vi "PathPlanner_Trajectory_CalculateVelocity.vi"(9 "MaxAccel":dbl, 10 "PathPoints":T1[](array[typedef]) {"HolonomicRotation"."SIN" format="%13.4f"; "HolonomicRotation"."COS" format="%13.4f"; "HolonomicRotation"."VALUE" format="%13.4f"; "NextControl"."Y" format="%14.3f"; "NextControl"."X" format="%14.3f"; "PrevControl"."Y" format="%14.3f"; "PrevControl"."X" format="%14.3f"; "AnchorPoint"."Y" format="%14.3f"; "AnchorPoint"."X" format="%14.3f"}, 11 "PathPlannerStates":T4[](array[typedef]) {"HolonomicRotation"."SIN" format="%13.4f"; "HolonomicRotation"."COS" format="%13.4f"; "HolonomicRotation"."VALUE" format="%13.4f"; "AngularVelocity"."SIN" format="%13.4f"; "AngularVelocity"."COS" format="%13.4f"; "AngularVelocity"."VALUE" format="%13.4f"; "TrajectoryState"."POSE"."ROTATION"."SIN" format="%13.4f"; "TrajectoryState"."POSE"."ROTATION"."COS" format="%13.4f"; "TrajectoryState"."POSE"."ROTATION"."VALUE" format="%13.4f"; "TrajectoryState"."POSE"."TRANSLATION"."Y" format="%14.3f"; "TrajectoryState"."POSE"."TRANSLATION"."X" format="%14.3f"; "AngularAcceleration"."SIN" format="%13.4f"; "AngularAcceleration"."COS" format="%13.4f"; "AngularAcceleration"."VALUE" format="%13.4f"}) -> (3 "outPathPlannerStates":T4[](array[typedef]) {"HolonomicRotation"."SIN" format="%13.4f"; "HolonomicRotation"."COS" format="%13.4f"; "HolonomicRotation"."VALUE" format="%13.4f"; "AngularVelocity"."SIN" format="%13.4f"; "AngularVelocity"."COS" format="%13.4f"; "AngularVelocity"."VALUE" format="%13.4f"; "TrajectoryState"."POSE"."ROTATION"."SIN" format="%13.4f"; "TrajectoryState"."POSE"."ROTATION"."COS" format="%13.4f"; "TrajectoryState"."POSE"."ROTATION"."VALUE" format="%13.4f"; "TrajectoryState"."POSE"."TRANSLATION"."Y" format="%14.3f"; "TrajectoryState"."POSE"."TRANSLATION"."X" format="%14.3f"; "AngularAcceleration"."SIN" format="%13.4f"; "AngularAcceleration"."COS" format="%13.4f"; "AngularAcceleration"."VALUE" format="%13.4f"})   [LabVIEW 2019, in "PathPlanner.lvlib"]
uses:
  PathPlanner.lvlib
  PathPlannerState.ctl
  <vilib>/Rock Robotics/WPI/ThirdParty/JAS_Junk/TrajLib/ROTATION2D.ctl
  <vilib>/Rock Robotics/WPI/ThirdParty/JAS_Junk/TrajLib/TRAJ_STATE.ctl
  <vilib>/Rock Robotics/WPI/ThirdParty/JAS_Junk/TrajLib/POSE2D.ctl
  <vilib>/Rock Robotics/WPI/ThirdParty/JAS_Junk/TrajLib/TRANSLATION2D.ctl
  PathPlannerWaypoint.ctl
  <vilib>/Rock Robotics/WPI/ThirdParty/JAS_Junk/TrajLib/Trajectory_Library.lvlib
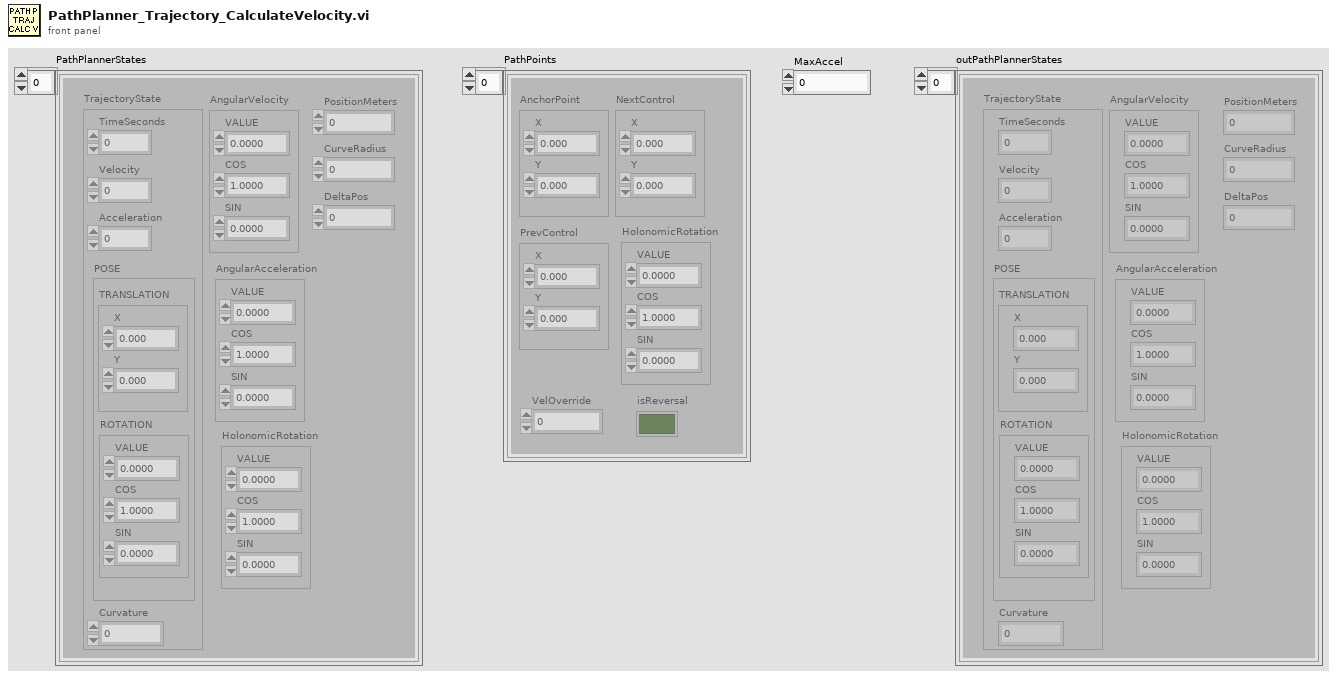
[diagram p1: front panel]
types:
  T1 = typedef "PathPlanner.lvlib/PathPlannerWaypoint.ctl" = cluster{"AnchorPoint":T2, "PrevControl":T2, "NextControl":T2, "HolonomicRotation":T3, "VelOverride":dbl, "isReversal":bool}
  T2 = typedef "Trajectory_Library.lvlib/TRANSLATION2D.ctl" = cluster{"X":dbl, "Y":dbl}
  T3 = typedef "Trajectory_Library.lvlib/ROTATION2D.ctl" = cluster{"VALUE":dbl, "COS":dbl, "SIN":dbl}
  T4 = typedef "PathPlanner.lvlib/PathPlannerState.ctl" = cluster{"AngularAcceleration":T3, "PositionMeters":dbl, "TrajectoryState":T5, "AngularVelocity":T3, "HolonomicRotation":T3, "CurveRadius":dbl, "DeltaPos":dbl}
  T5 = typedef "Trajectory_Library.lvlib/TRAJ_STATE.ctl" = cluster{"TimeSeconds":dbl, "Velocity":dbl, "Acceleration":dbl, "POSE":T6, "Curvature":dbl}
  T6 = typedef "Trajectory_Library.lvlib/POSE2D.ctl" = cluster{"TRANSLATION":T2, "ROTATION":T3}
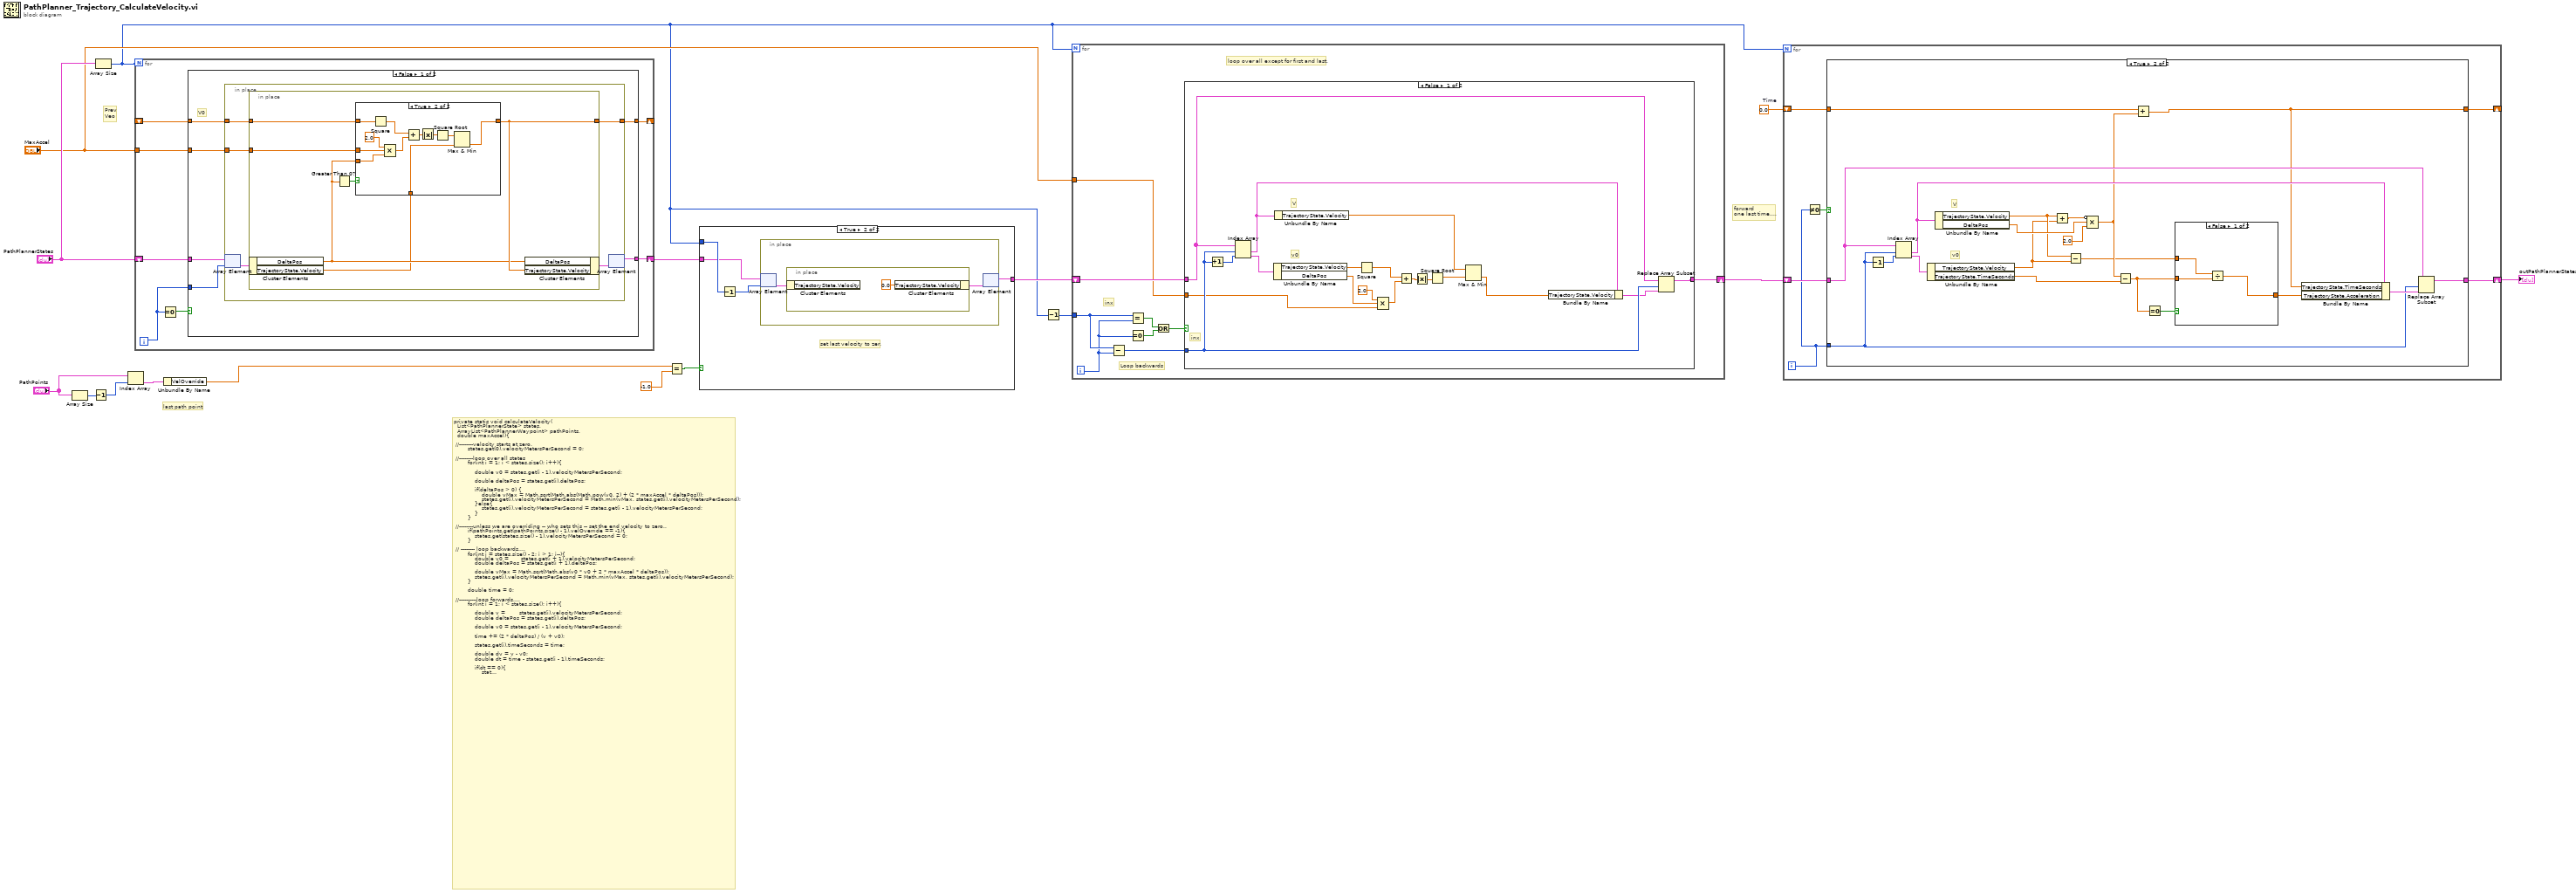
[diagram p0: block diagram]
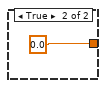
[diagram p3: hidden frame]
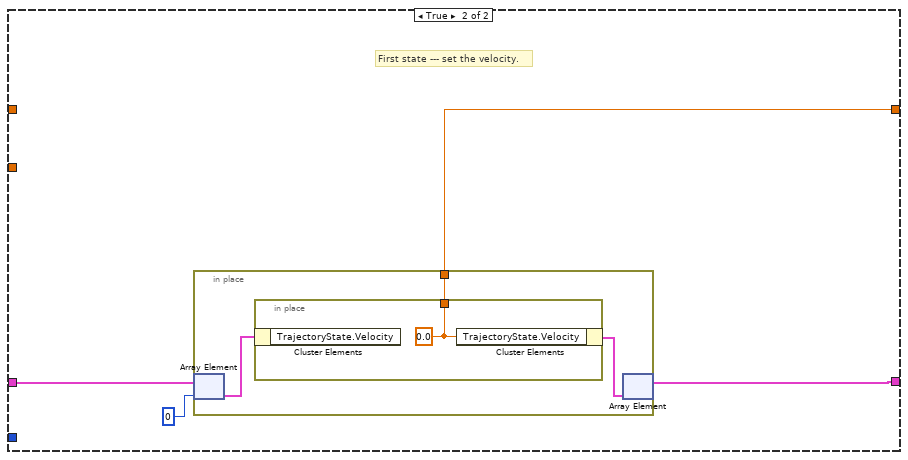
[diagram p7: hidden frame]
diagram:
  w4 = 0.0  # Time
  # "last path point"
  # "private static void calculateVelocity(\n\t\tList<PathPlannerState> states, \n\t\tArrayList<PathPlannerWaypoint> pathPoints, \n\t\tdouble maxAccel){\n\n\t//--------velocity starts at zero.\n        states.get(0).velocityMetersPerSecond = 0;\n\n\t//--------loop over all states\n        for(int i = 1; i < states.size(); i++){\n\n            double v0 = states.get(i - 1).velocityMetersPerSecond;\n\n            double deltaPos = states.get(i).deltaPos;\n\n            if(deltaPos > 0) {\n                double vMax = Math.sqrt(Math.abs(Math.pow(v0, 2) + (2 * maxAccel * deltaPos)));\n                states.get(i).velocityMetersPerSecond = Math.min(vMax, states.get(i).velocityMetersPerSecond);\n            }else{\n                states.get(i).velocityMetersPerSecond = states.get(i - 1).velocityMetersPerSecond;\n            }\n        }\n\n\t//--------unless we are overriding -- who sets this -- set the end velocity to zero..\n        if(pathPoints.get(pathPoints.size() - 1).velOverride == -1){\n            states.get(states.size() - 1).velocityMetersPerSecond = 0;\n        }\n\n\t// -------- loop backwards....\n        for(int i = states.size() - 2; i > 1; i--){\n            double v0 =       states.get(i + 1).velocityMetersPerSecond;\n            double deltaPos = states.get(i + 1).deltaPos;\n\n            double vMax = Math.sqrt(Math.abs(v0 * v0 + 2 * maxAccel * deltaPos));\n            states.get(i).velocityMetersPerSecond = Math.min(vMax, states.get(i).velocityMetersPerSecond);\n        }\n\n        double time = 0;\n\n\t//----------loop forwards....\n        for(int i = 1; i < states.size(); i++){\n\n            double v =        states.get(i).velocityMetersPerSecond;\n            double deltaPos = states.get(i).deltaPos;\n\n            double v0 = states.get(i - 1).velocityMetersPerSecond;\n\n            time += (2 * deltaPos) / (v + v0);\n\n            states.get(i).timeSeconds = time;\n\n            double dv = v - v0;\n            double dt = time - states.get(i - 1).timeSeconds;\n\n            if(dt == 0){\n                states.get(i).accelerationMetersPerSecondSq = 0;\n            }else{\n                states.get(i).accelerationMetersPerSecondSq = dv / dt;\n            }\n        }\n    }"
  # "forward\none last time...."
  # "Prev\nVeo"
  n1 = Array Size(array="PathPoints") -> (size(s)=w15:i32)
  n2 = Decrement(x=w15) -> (x-1=w13:i32)
  n3 = Array Size(array="PathPlannerStates") -> (size(s)=w1:i32)
  n4 = Index Array(array="PathPoints", index=w13) -> (element=w12:T1)
  n5 = for {
    N: w1 -> [_]
    shift-right: [w21] -> w8
    shift-left: "PathPlannerStates" -> [w22]
    shift-right: [w20] -> _
    shift-left: _ -> [w18]
    tunnel: "MaxAccel" -> [w17]
    i -> [w19]
    n6 = Equal To 0?(x=w19) -> (x = 0?=w23:bool)
    n7 = case shown="False" w23 {
      tunnel: w22 -> [w26 w56]
      tunnel: [w24 w55] -> w21
      tunnel: [w28 w53] -> w20
      tunnel: w19 -> [w25 _]
      tunnel: w18 -> [w29 _]
      tunnel: w17 -> [w27 _]
      frame False {
        # "V0"
        n8 = in-place {
          in-place-border: w29 -> [w34]
          in-place-border: [w33] -> w28
          in-place-border: w27 -> [w32]
          n9 = in-place-array #1(w26, w25) -> (w31:T4)
          n10 = in-place {
            in-place-border: w34 -> [w39]
            in-place-border: [w38] -> w33
            in-place-border: w32 -> [w37]
            n11 = in-place-cluster #2(w31) -> ("DeltaPos"=w36:dbl, "TrajectoryState.Velocity"=w35:dbl)
            n12 = Greater Than 0?(x=w36) -> (x > 0?=w40:bool)
            n13 = case shown="True" w40 {
              tunnel: w39 -> [w41 w52]
              tunnel: [w41 w44] -> w38
              tunnel: w37 -> [_ w50]
              tunnel: w36 -> [_ w49]
              tunnel: w35 -> [_ w45]
              frame False {
              }
              frame True {
                n14 = Square(x=w52) -> (x^2=w48:dbl)
                n15 = Compound Arithmetic op=MULTIPLY(2.0 ("value"), w50, w49) -> (w47:dbl)
                n16 = Add(x=w48, y=w47) -> (x+y=w42:dbl)
                n17 = Absolute Value(x=w42) -> (abs(x)=w43:dbl)
                n18 = Square Root(x=w43) -> (sqrt(x)=w46:dbl)
                n19 = Max & Min(x=w46, y=w45) -> (min(x,y)=w44:dbl)  [unwired: 1 out]
              }
            }
            n20 = in-place-cluster #2("DeltaPos"=w36, "TrajectoryState.Velocity"=w38) -> (w30:T4)
          }
          n21 = in-place-array #1(w30) -> (w24:T4[])  [unwired: 1 out]
        }
      }
      frame True {
        # "First state --- set the velocity."
        n22 = in-place {
          in-place-border: [w57] -> w53
          n23 = in-place-array #3(w56, 0) -> (w59:T4)
          n24 = in-place {
            in-place-border: [w60] -> w57
            w60 = 0.0 ("TrajectoryState.Velocity")
            n25 = in-place-cluster #4(w59) -> ()  [unwired: 1 out]
            n26 = in-place-cluster #4("TrajectoryState.Velocity"=w60) -> (w58:T4)
          }
          n27 = in-place-array #3(w58) -> (w55:T4[])  [unwired: 1 out]
        }
      }
    }
  }
  n28 = Unbundle By Name(w12) -> ("VelOverride"=w9:dbl)
  n29 = Equal?(x=w9, y=-1.0) -> (x = y?=w11:bool)
  n30 = case shown="True" w11 {
    tunnel: w8 -> [w61 w64]
    tunnel: w1 -> [_ w65]
    tunnel: [w61 w63] -> w7
    frame False {
    }
    frame True {
      # "set last velocity to zer."
      n31 = Decrement(x=w65) -> (x-1=w62:i32)
      n32 = in-place {
        n33 = in-place-array #5(w64, w62) -> (w67:T4)
        n34 = in-place {
          n35 = in-place-cluster #6(w67) -> ()  [unwired: 1 out]
          n36 = in-place-cluster #6("TrajectoryState.Velocity"=0.0) -> (w66:T4)
        }
        n37 = in-place-array #5(w66) -> (w63:T4[])  [unwired: 1 out]
      }
    }
  }
  n38 = Decrement(x=w1) -> (x-1=w6:i32)
  n39 = for {
    N: w1 -> [_]
    shift-right: [w71] -> w5
    shift-left: w7 -> [w72]
    tunnel: w6 -> [w77]
    tunnel: "MaxAccel" -> [w70]
    i -> [w69]
    # "loop over all except for first and last."
    # "inx"
    # "Loop backwards"
    n40 = Subtract(x=w77, y=w69) -> (x-y=w73:i32)
    n41 = Equal?(x=w77, y=w69) -> (x = y?=w76:bool)
    n42 = Equal To 0?(x=w69) -> (x = 0?=w75:bool)
    n43 = Or(x=w76, y=w75) -> (x .or. y?=w74:bool)
    n44 = case shown="False" w74 {
      tunnel: w73 -> [w90 _]
      tunnel: w72 -> [w91 w96]
      tunnel: [w93 w96] -> w71
      tunnel: w70 -> [w85 _]
      frame False {
        # "v0"
        # "V"
        # "inx"
        n45 = Increment(x=w90) -> (x+1=w95:i32)
        n46 = Index Array(array=w91, index #1=w90, index #2=w95) -> (element #1=w92:T4, element #2=w94:T4)
        n47 = Unbundle By Name(w94) -> ("TrajectoryState.Velocity"=w88:dbl, "DeltaPos"=w86:dbl)
        n48 = Unbundle By Name(w92) -> ("TrajectoryState.Velocity"=w80:dbl)
        n49 = Square(x=w88) -> (x^2=w84:dbl)
        n50 = Compound Arithmetic op=MULTIPLY(2.0 ("value"), w86, w85) -> (w83:dbl)
        n51 = Add(x=w84, y=w83) -> (x+y=w79:dbl)
        n52 = Absolute Value(x=w79) -> (abs(x)=w78:dbl)
        n53 = Square Root(x=w78) -> (sqrt(x)=w82:dbl)
        n54 = Max & Min(x=w80, y=w82) -> (min(x,y)=w81:dbl)  [unwired: 1 out]
        n55 = Bundle By Name(cluster=w92, "TrajectoryState.Velocity"=w81) -> (w89:T4)
        n56 = Replace Array Subset(array=w91, new element=w89, index=w90) -> (w93:T4[])
      }
      frame True {
        # "For first and last states, do nothing."
      }
    }
  }
  n57 = for {
    N: w1 -> [_]
    shift-right: [w101] -> w2
    shift-left: w5 -> [w102]
    shift-right: [w99] -> _
    shift-left: w4 -> [w100]
    i -> [w97]
    n58 = Not Equal To 0?(x=w97) -> (x != 0?=w98:bool)
    n59 = case shown="True" w98 {
      tunnel: w102 -> [w103 w124]
      tunnel: [w103 w123] -> w101
      tunnel: w100 -> [w104 w115]
      tunnel: [w104 w105] -> w99
      tunnel: w97 -> [_ w106]
      frame False {
        # "first time.... do nothing..."
      }
      frame True {
        # "v0"
        # "V"
        n60 = Decrement(x=w106) -> (x-1=w122:i32)
        n61 = Index Array(array=w124, index #1=w106, index #2=w122) -> (element #1=w120:T4, element #2=w121:T4)
        n62 = Unbundle By Name(w121) -> ("TrajectoryState.Velocity"=w113:dbl, "TrajectoryState.TimeSeconds"=w112:dbl)
        n63 = Unbundle By Name(w120) -> ("TrajectoryState.Velocity"=w114:dbl, "DeltaPos"=w117:dbl)
        n64 = Add(x=w114, y=w113) -> (x+y=w118:dbl)
        n65 = Subtract(x=w114, y=w113) -> (x-y=w108:dbl)
        n66 = Compound Arithmetic op=MULTIPLY(invert w118, w117, 2.0 ("value")) -> (w111:dbl)
        n67 = Subtract(x=w111, y=w112) -> (x-y=w107:dbl)
        n68 = Add(x=w115, y=w111) -> (x+y=w105:dbl)
        n69 = Equal To 0?(x=w107) -> (x = 0?=w110:bool)
        n70 = case shown="False" w110 {
          tunnel: [w125 0.0] -> w109
          tunnel: w108 -> [w127 _]
          tunnel: w107 -> [w126 _]
          frame False {
            n71 = Divide(x=w127, y=w126) -> (x/y=w125:dbl)
          }
          frame True {
          }
        }
        n72 = Bundle By Name(cluster=w120, "TrajectoryState.TimeSeconds"=w105, "TrajectoryState.Acceleration"=w109) -> (w119:T4)
        n73 = Replace Array Subset(array=w124, new element=w119, index=w106) -> (w123:T4[])
      }
    }
  }
  "outPathPlannerStates" <- w2
